vi "Change Representation.vi"(8 "error in (no error)":errorcluster, 10 "Representation":T1, 11 "Numeric Data Type in":refnum<class "Numeric Data Type.lvclass">) -> (0 "error out":errorcluster, 3 "Numeric Data Type out":refnum<class "Numeric Data Type.lvclass">)   [LabVIEW 2018, in "Numeric Data Type.lvclass"]
uses:
  Numeric Data Type.lvclass
  Representation Ring.ctl
  Numeric Data Type.lvclass/Numeric Data Type.ctl
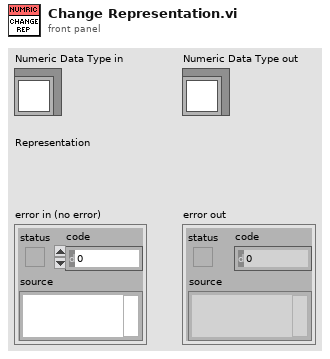
[diagram p1: front panel]
types:
  T1 = typedef "Numeric Data Type.lvclass/Representation Ring.ctl" = u16
  T2 = typedef "Numeric Data Type.lvclass/Representation Enum.ctl" = enum16{"Extended (EXT)", "Double (DBL)", "Single (SGL)", "Fixed-Point (FXP)", "Quad Integer (I64)", "Long Integer (I32)", "Word Integer (I16)", "Byte Integer (I8)", "Unsigned Quad (U64)", "Unsigned Long (U32)", "Unsigned Word (U16)", "Unsigned Byte (U8)", "Complex Extended (CXT)", "Complex Double (CDB)", "Complex Single (CSG)"}
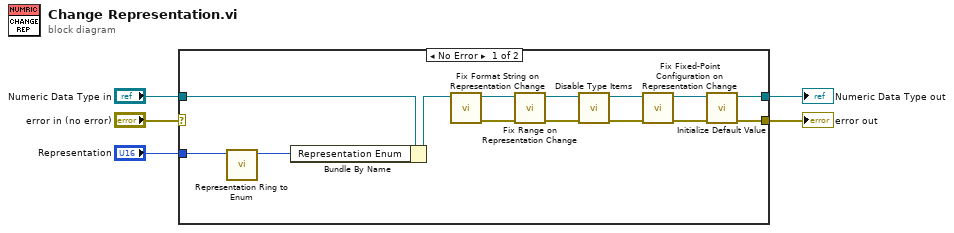
[diagram p0: block diagram]
diagram:
  n1 = case shown="No Error" "error in (no error)" {
    selector: "error in (no error)" -> [_ w21]
    tunnel: [w6 w21] -> w4
    tunnel: [w7 w20] -> w2
    tunnel: "Numeric Data Type in" -> [w18 w20]
    tunnel: "Representation" -> [w19 _]
    frame No Error {
      n2 = call "Representation Ring to Enum.vi"("Representation Ring"=w19) -> ("Representation Enum"=w17:T2)  [unwired: 10 in]
      n3 = Bundle By Name(cluster=w18, "Representation Enum"=w17) -> (w12:refnum<class "Numeric Data Type.lvclass">)
      n4 = call "Fix Format String on Representation Change.vi"("Numeric Data Type in"=w12) -> ("error out"=w10:errorcluster, "Numeric Data Type out"=w11:refnum<class "Numeric Data Type.lvclass">)  [unwired: 9 in]
      n5 = call "Fix Range on Representation Change.vi"("error in (no error)"=w10, "Numeric Data Type in"=w11) -> ("error out"=w14:errorcluster, "Numeric Data Type out"=w15:refnum<class "Numeric Data Type.lvclass">)  [unwired: 8 in]
      n6 = call "Disable Type Items.vi"("error in (no error)"=w14, "Numeric Data Type in"=w15) -> ("error out"=w16:errorcluster, "Numeric Data Type out"=w13:refnum<class "Numeric Data Type.lvclass">)  [unwired: 8 in]
      n7 = call "Fix Fixed-Point Configuration on Representation Change.vi"("error in (no error)"=w16, "Numeric Data Type in"=w13) -> ("error out"=w8:errorcluster, "Numeric Data Type out"=w9:refnum<class "Numeric Data Type.lvclass">)  [unwired: 8 in]
      n8 = call "Initialize Default Value.vi"("error in (no error)"=w8, "Numeric Data Type in"=w9) -> ("error out"=w6:errorcluster, "Numeric Data Type (dup)"=w7:refnum<class "Numeric Data Type.lvclass">)  [unwired: 8 in]
    }
    frame Error {
    }
  }
  "error out" <- w4
  "Numeric Data Type out" <- w2
